vi "Signal Filter.vi"(10 "Y PWM FPGA":dbl, 11 "X PWM FPGA":dbl) -> (2 "Y PWM Out":dbl, 3 "X PWM Out":dbl)   [LabVIEW 2015]
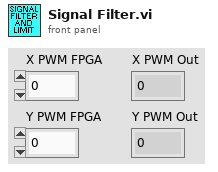
[diagram p1: front panel]
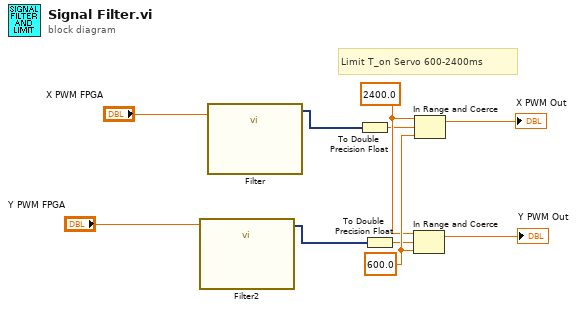
[diagram p0: block diagram]
diagram:
  w8 = 600.0 ("upper limit")
  w7 = 2400.0 ("upper limit")
  # "Limit T_on Servo 600-2400ms"
  n1 = call "Filter2"("Signal"="Y PWM FPGA") -> ("Filtered Signal"=w2:dynamicdata)  [unwired: 9 in, 1 out]
  n2 = call "Filter"("Signal"="X PWM FPGA") -> ("Filtered Signal"=w1:dynamicdata)  [unwired: 9 in, 1 out]
  n3 = To Double Precision Float(number=w1) -> (double precision float=w5:dbl)
  n4 = To Double Precision Float(number=w2) -> (double precision float=w6:dbl)
  n5 = In Range and Coerce(upper limit=w7, x=w6, lower limit=w8) -> (coerced(x)=→"Y PWM Out":dbl)  [unwired: 1 out]
  n6 = In Range and Coerce(upper limit=w7, x=w5, lower limit=w8) -> (coerced(x)=→"X PWM Out":dbl)  [unwired: 1 out]
